vi "get_display_data.vi"(5 "Modulation info":T14 {"Hi channels at low" min=0 step=1; "Low carriers" format="%#_6p"; "High carriers" format="%#_6p"}, 10 "Trace info":T2, 11 "Display options":T5 {"Spectrum parameters"."Order" min=1 max=100; "Spectrum parameters"."Averaging" min=0.0 max=1000.0 step=1.0}) -> (1 "Sample rate":dbl, 2 "Demodulated signal":T1 format="%#_3p", 3 "Time signal":dbl[][](array[numeric]), 4 "Chart data?":bool, 6 "Demodulated?":bool)   [LabVIEW 2026]
uses:
  processing/modulation_info.ctl
  display_options.ctl
  display_source.ctl
  axis_name.ctl
  spectrum_parameters.ctl
  levels_selector.ctl
  Level selector 1.ctl
  Level selector 4.ctl
  Level selector 3.ctl
  Level selector 2.ctl
  trace_info.ctl
  trace_channel.ctl
  main/ilemt_status.ctl
  processing/card_high_carrier_amplitudes.ctl
  <vilib>/Analysis/2dsp.llb/Inverse Real FFT.vi
  <vilib>/Analysis/NI_AALPro.lvlib
panel:
  # "In channel"
  # "Sample"
  # "The output sample rate."
  # "Is this a demodulated complex signal?"
  # "Used for chart data, where successive outputs are overlapping"
  # "Extract signal data from a \"Trace info\", according to \"Display options\".  Sometimes the signal is a real time-domain signal, and sometimes it is a demodulated complex frequency/time signal.  For a complex signal, we generate a time signal by taking magnitude or phase of the samples.  If the signal is real, then \"Demodulated?\" is false, and \"Demodulated signal\" is empty."
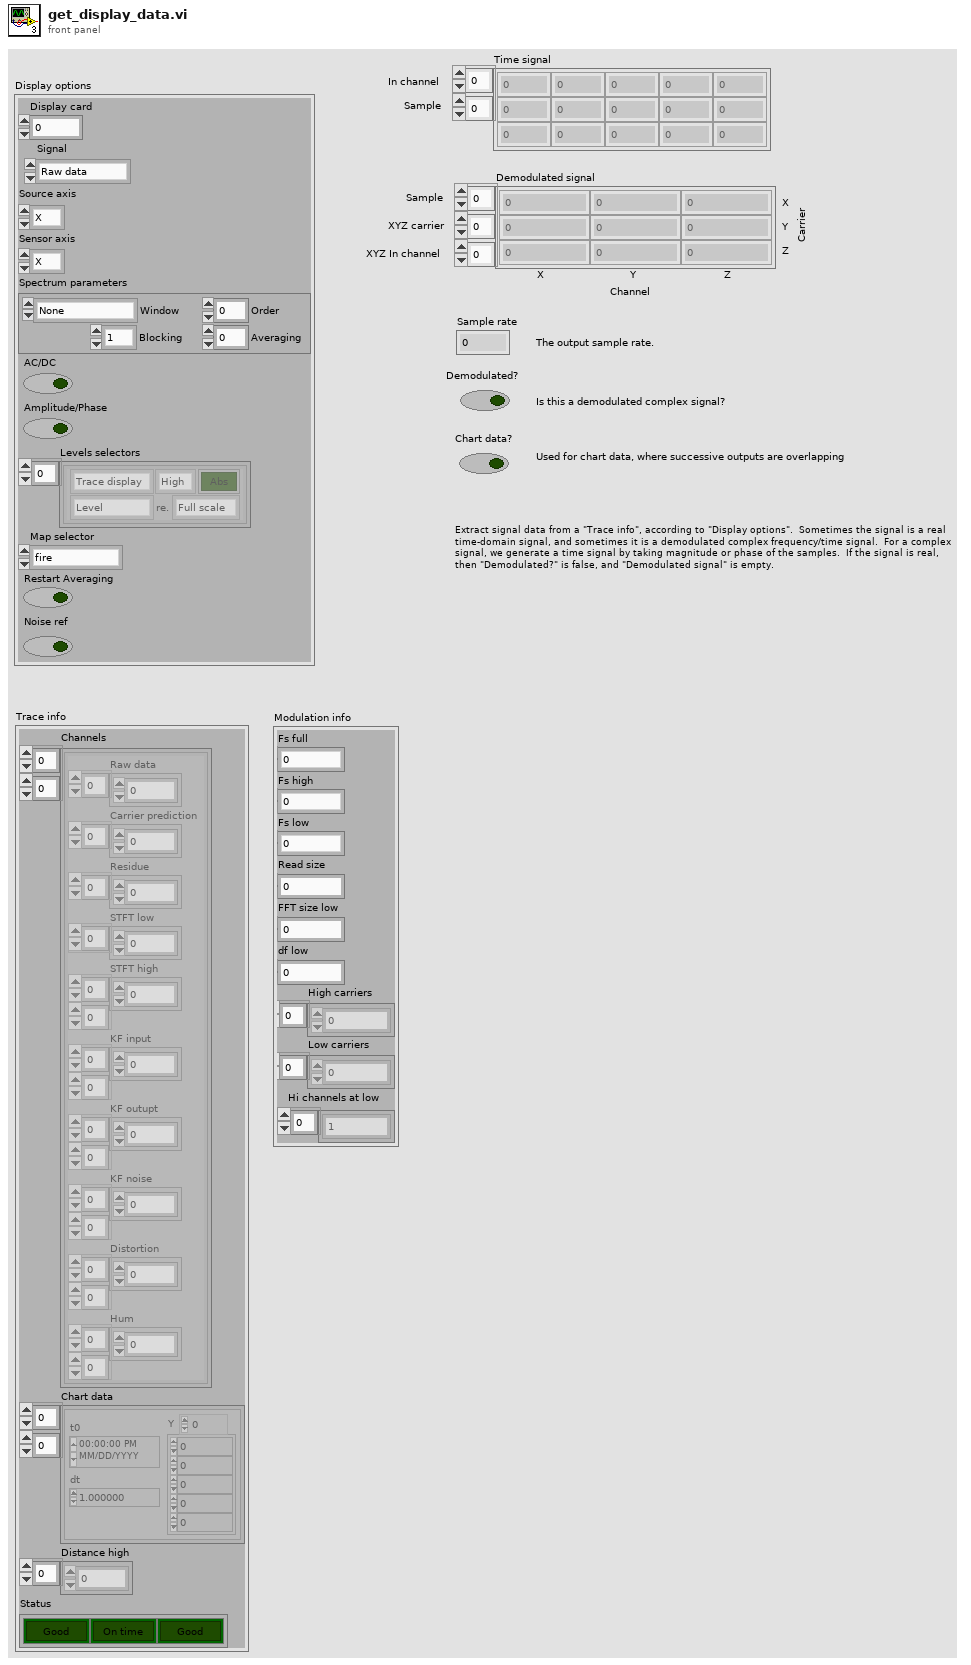
[diagram p1: front panel]
types:
  T1 = typedef "card_high_carrier_amplitudes.ctl" = cdb[][][]
  T2 = typedef "trace_info.ctl" = cluster{"Channels":T3[][], "Chart data":waveform(dbl)[][], "Distance high":dbl[], "Status":T4}
  T3 = typedef "trace_channel.ctl" = cluster{"Raw data":dbl[], "Carrier prediction":dbl[], "Residue":dbl[], "STFT low":cdb[], "STFT high":cdb[][], "KF input":cdb[][], "KF outupt":cdb[][], "KF noise":dbl[][], "Distortion":cdb[][], "Hum":cdb[][]}
  T4 = typedef "ilemt_status.ctl" = cluster{"NaN":bool, "Backlog":bool, "Clipping":bool}
  T5 = typedef "display_options.ctl" = cluster{"Display card":i32, "Signal":T6, "Source axis":T7, "Sensor axis":T7, "Spectrum parameters":T8, "AC/DC":bool, "Amplitude/Phase":bool, "Levels selectors":T9[], "Map selector":enum16{"fire", "rainbow", "grey", "inverse grey", "ice", "original"}, "Restart Averaging":bool, "Noise ref":bool}
  T6 = typedef "display_source.ctl" = enum16{"Raw data", "Carrier predict", "Residue", "STFT low", "STFT high", "KF input", "KF output", "KF noise", "Distortion", "Hum", "Distance high", "Chart high", "Chart low"}
  T7 = typedef "axis_name.ctl" = enum16{"X", "Y", "Z"}
  T8 = typedef "spectrum_parameters.ctl" = cluster{"Window":enum16{"None ", "Hanning", "Hamming", "Blackman-Harris", "Exact Blackman", "Blackman", "Flat Top", "4 Term B-Harris ", "7 Term B-Harris", "Low Sidelobe"}, "FFT blocking":enum16{"1", "2", "4", "8"}, "Averaging":dbl, "Order":u32}
  T9 = typedef "levels_selector.ctl" = cluster{"Signal source":T10, "Mode":T11, "re.":T12, "High/low":T13, "Sense":bool}
  T10 = typedef "Level selector 1.ctl" = enum16{"Trace display", "Carrier levels", "Ref levels"}
  T11 = typedef "Level selector 4.ctl" = enum16{"Level", "dB", "Phase", "Mismatch"}
  T12 = typedef "Level selector 3.ctl" = enum16{"Full scale", "Carrier", "Ref level", "Noise"}
  T13 = typedef "Level selector 2.ctl" = enum16{"High", "Low"}
  T14 = typedef "modulation_info.ctl" = cluster{"Fs full":dbl, "Fs high":dbl, "Fs low":dbl, "Read size":i32, "FFT size low":i32, "df low":dbl, "High carriers":dbl[], "Low carriers":dbl[], "Hi channels at low":i32[]}
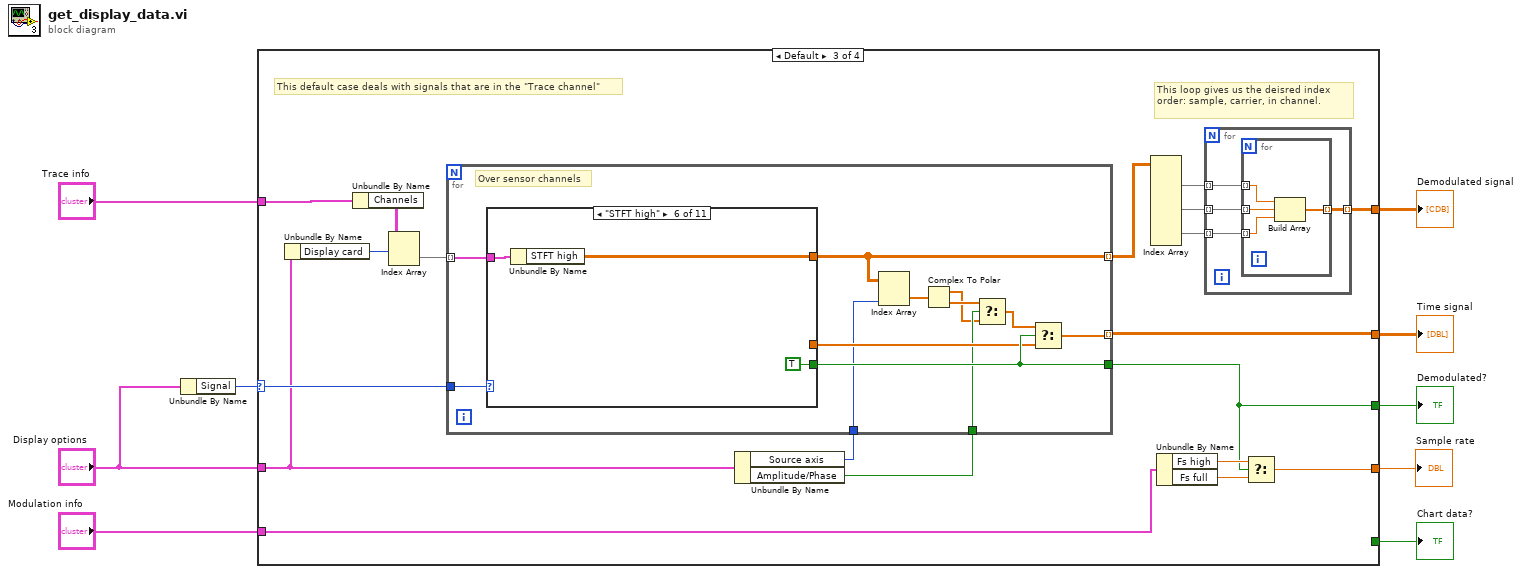
[diagram p0: block diagram]
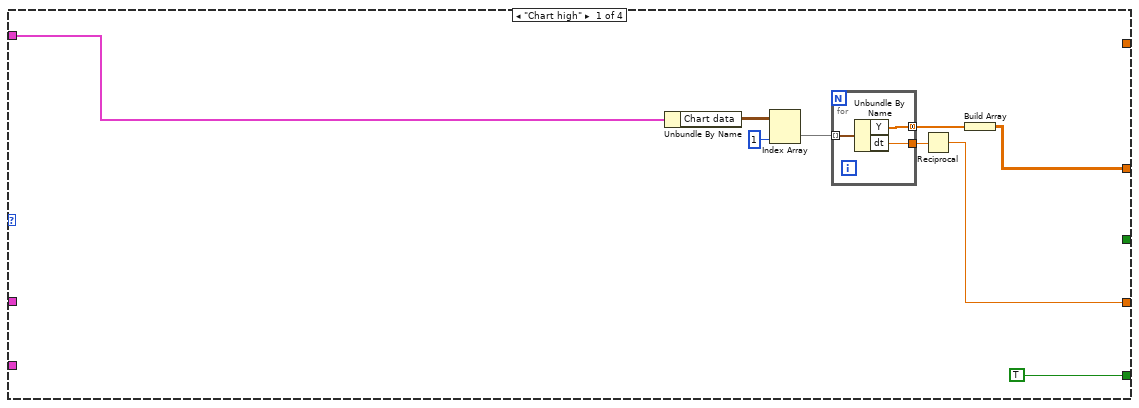
[diagram p2: hidden frame]
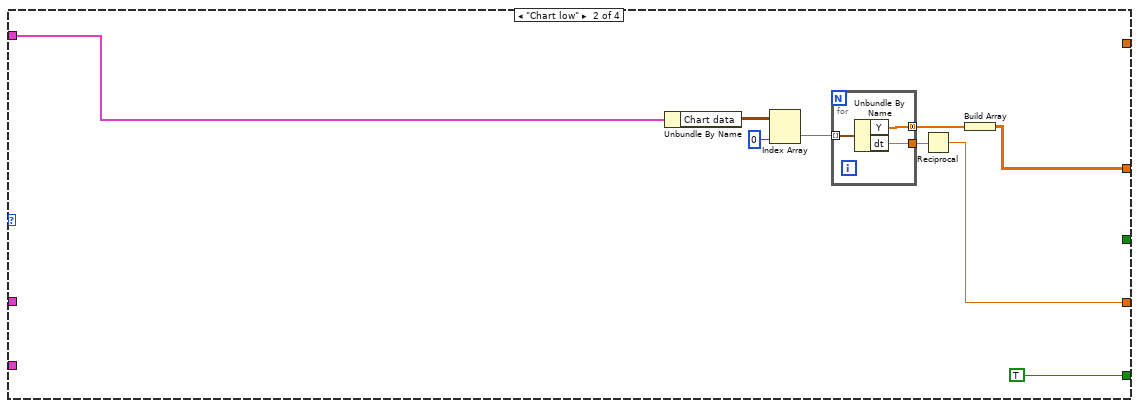
[diagram p3: hidden frame]
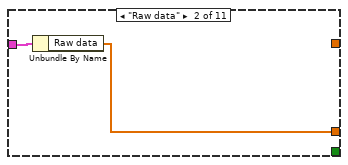
[diagram p5: hidden frame]
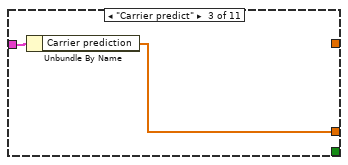
[diagram p6: hidden frame]
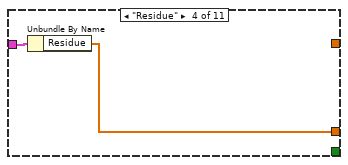
[diagram p7: hidden frame]
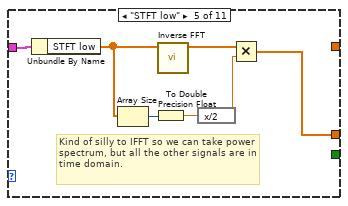
[diagram p8: hidden frame]
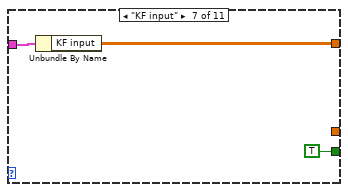
[diagram p9: hidden frame]
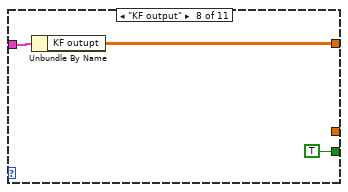
[diagram p10: hidden frame]
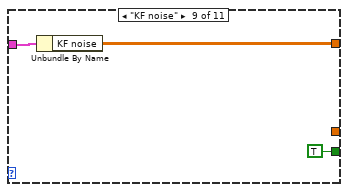
[diagram p11: hidden frame]
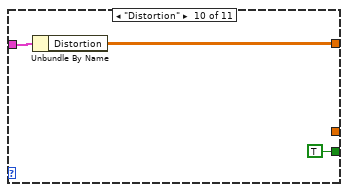
[diagram p12: hidden frame]
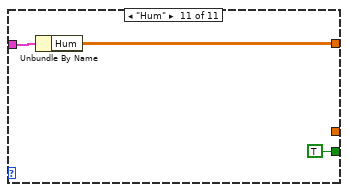
[diagram p13: hidden frame]
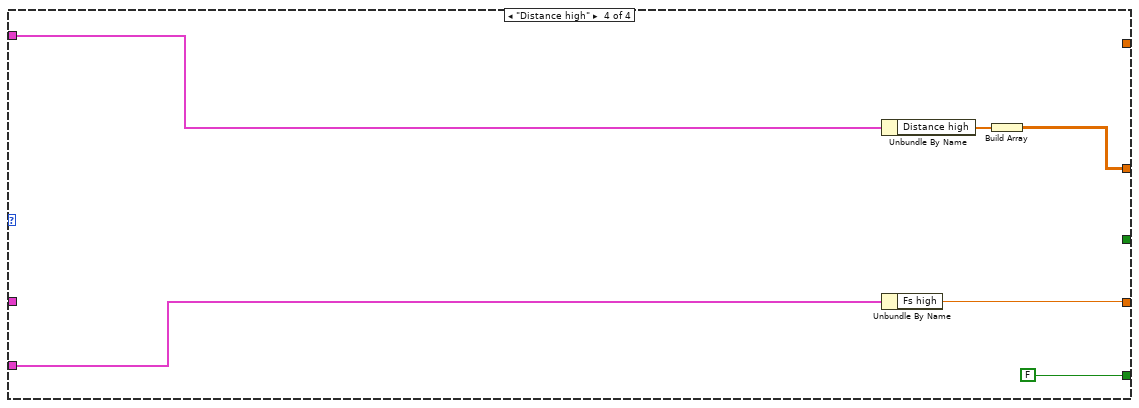
[diagram p14: hidden frame]
diagram:
  n1 = Unbundle By Name("Display options") -> ("Signal"=w6:T6)
  n2 = case shown="Default" w6 {
    selector: w6 -> [_ _ w51 _]
    tunnel: "Trace info" -> [w14 w26 w52 w108]
    tunnel: [w12 w24 w34 w106] -> w7
    tunnel: "Modulation info" -> [_ _ w48 w109]
    tunnel: [_ _ w35 _] -> w5
    tunnel: [_ _ w44 _] -> w4
    tunnel: [w10 w22 w45 w104] -> w3
    tunnel: [TRUE ("Demodulated?") TRUE ("Demodulated?") _ FALSE ("Demodulated?")] -> w2
    tunnel: "Display options" -> [_ _ w42 _]
    frame "Chart high" {
      n3 = Unbundle By Name(w14) -> ("Chart data"=w18:waveform(dbl)[][])
      n4 = Index Array(array=w18, index (col)=1 ("index (row)")) -> (element=w17:waveform(dbl)[])  [unwired: 1 in]
      n5 = for {
        tunnel: w17 -> [w21] mode=indexing
        tunnel: [w20] -> w13 mode=concatenating
        tunnel: [w19] -> w15
        n6 = Unbundle By Name(w21) -> ("Y"=w20:dbl[], "dt"=w19:dbl)
      }
      n7 = Reciprocal(x=w15) -> (1/x=w10:dbl)
      n8 = Build Array(w13) -> (w12:dbl[][])
    }
    frame "Chart low" {
      n9 = Unbundle By Name(w26) -> ("Chart data"=w30:waveform(dbl)[][])
      n10 = Index Array(array=w30, index (col)=0 ("index (row)")) -> (element=w29:waveform(dbl)[])  [unwired: 1 in]
      n11 = for {
        tunnel: w29 -> [w33] mode=indexing
        tunnel: [w32] -> w25 mode=concatenating
        tunnel: [w31] -> w27
        n12 = Unbundle By Name(w33) -> ("Y"=w32:dbl[], "dt"=w31:dbl)
      }
      n13 = Reciprocal(x=w27) -> (1/x=w22:dbl)
      n14 = Build Array(w25) -> (w24:dbl[][])
    }
    frame Default {
      # "This loop gives us the deisred index order: sample, carrier, in channel."
      # "This default case deals with signals that are in the \"Trace channel\""
      n15 = Unbundle By Name(w42) -> ("Display card"=w43:i32)
      n16 = Unbundle By Name(w52) -> ("Channels"=w50:T3[][])
      n17 = Index Array(array=w50, index (row)=w43) -> (element=w49:T3[])  [unwired: 1 in]
      n18 = Unbundle By Name(w42) -> ("Source axis"=w41:T7, "Amplitude/Phase"=w40:bool)
      n19 = for {
        tunnel: [w62] -> w34 mode=indexing
        tunnel: w51 -> [w71]
        tunnel: w49 -> [w72] mode=indexing
        tunnel: [w69] -> w39 mode=indexing
        tunnel: [w70] -> w44
        tunnel: w41 -> [w61]
        tunnel: w40 -> [w66]
        # "Over sensor channels"
        n20 = case shown="\"STFT high\"" w71 {
          tunnel: w72 -> [_ w74 w76 w78 w80 w88 w91 w94 w97 w100 w103]
          tunnel: [_ _ _ _ _ w87 w90 w93 w96 w99 w102] -> w69
          tunnel: [_ w73 w75 w77 w79 _ _ _ _ _ _] -> w68
          tunnel: [_ _ _ _ _ TRUE ("Demodulated?") TRUE ("Demodulated?") TRUE ("Demodulated?") TRUE ("Demodulated?") TRUE ("Demodulated?") TRUE ("Demodulated?")] -> w70
          frame Default {
          }
          frame "Raw data" {
            n21 = Unbundle By Name(w74) -> ("Raw data"=w73:dbl[])
          }
          frame "Carrier predict" {
            n22 = Unbundle By Name(w76) -> ("Carrier prediction"=w75:dbl[])
          }
          frame "Residue" {
            n23 = Unbundle By Name(w78) -> ("Residue"=w77:dbl[])
          }
          frame "STFT low" {
            # "Kind of silly to IFFT so we can take power spectrum, but all the other signals are in time domain."
            n24 = Unbundle By Name(w80) -> ("STFT low"=w85:cdb[])
            n25 = Array Size(array=w85) -> (size(s)=w82:i32)
            n26 = To Double Precision Float(number=w82) -> (double precision float=w81:dbl)
            n27 = call-poly <vilib>:"Inverse FFT.vi"("FFT {X}"=w85) -> ("X"=w83:dbl[])  [unwired: 9 in, 1 out]
            n28 = expression code="x/2"(w81) -> (w84:dbl)
            n29 = Multiply(x=w83, y=w84) -> (x*y=w79:dbl[])
          }
          frame "STFT high" {
            n30 = Unbundle By Name(w88) -> ("STFT high"=w87:cdb[][])
          }
          frame "KF input" {
            n31 = Unbundle By Name(w91) -> ("KF input"=w90:cdb[][])
          }
          frame "KF output" {
            n32 = Unbundle By Name(w94) -> ("KF outupt"=w93:cdb[][])
          }
          frame "KF noise" {
            n33 = Unbundle By Name(w97) -> ("KF noise"=w96:dbl[][])
          }
          frame "Distortion" {
            n34 = Unbundle By Name(w100) -> ("Distortion"=w99:cdb[][])
          }
          frame "Hum" {
            n35 = Unbundle By Name(w103) -> ("Hum"=w102:cdb[][])
          }
        }
        n36 = Index Array(array=w69, index (col)=w61) -> (element=w67:cdb[])  [unwired: 1 in]
        n37 = Complex To Polar(r * e^(i*theta)=w67) -> (r=w64:dbl[], theta=w65:dbl[])
        n38 = Select(t=w65, s=w66, f=w64) -> (s? t:f=w63:dbl[])
        n39 = Select(t=w63, s=w70, f=w68) -> (s? t:f=w62:dbl[])
      }
      n40 = Index Array(array=w39) -> (element #1=w38:cdb[][], element #2=w37:cdb[][], element #3=w36:cdb[][])  [unwired: 9 in]
      n41 = Unbundle By Name(w48) -> ("Fs high"=w47:dbl, "Fs full"=w46:dbl)
      n42 = for {
        tunnel: w38 -> [w54] mode=indexing
        tunnel: w37 -> [w55] mode=indexing
        tunnel: w36 -> [w56] mode=indexing
        tunnel: [w53] -> w35 mode=indexing
        n43 = for {
          tunnel: w56 -> [w59] mode=indexing
          tunnel: w55 -> [w60] mode=indexing
          tunnel: w54 -> [w58] mode=indexing
          tunnel: [w57] -> w53 mode=indexing
          n44 = Build Array(w58, w60, w59) -> (w57:cdb[])
        }
      }
      n45 = Select(t=w47, s=w44, f=w46) -> (s? t:f=w45:dbl)
    }
    frame "Distance high" {
      n46 = Unbundle By Name(w108) -> ("Distance high"=w107:dbl[])
      n47 = Unbundle By Name(w109) -> ("Fs high"=w104:dbl)
      n48 = Build Array(w107) -> (w106:dbl[][])
    }
  }
  "Sample rate" <- w3
  "Time signal" <- w7
  "Demodulated signal" <- w5
  "Demodulated?" <- w4
  "Chart data?" <- w2
